vi "Test Host Image Acquisition Module Random Data.vi"(8 "error in":errorcluster, 11 "Operation":T3) -> (0 "error out":errorcluster, 1 "Image Acquired":bool, 2 "Acq In Progress":bool, 3 "Image":T2(plugin-control))   [LabVIEW 2013]
uses:
  Host/Image Acquisition/Host Image Acquisition Module Enum.ctl
  Host/Image Acquisition/Acquisition Settings Cluster.ctl
  <vilib>/vision/Image Controls.llb/IMAQ Image.ctl
  Host/Image Acquisition/Image Acquisition Settings FG Enum.ctl
  Host/System Status/Status FG Enum.ctl
  Host/Image Processing/Mask ROI FG Enum.ctl
  <vilib>/FPGAPlugInAG/PCIe-7842R/niLvFpga_Reset_PCIe-7842R.vi
  <vilib>/Utility/error.llb/Error Cluster From Error Code.vi
  <vilib>/rvi/errors/niLvFpgaAdjustHostInterfaceError.vi
  <vilib>/FPGAPlugInAG/PCIe-7842R/niLvFpga_Run_PCIe-7842R.vi
  <vilib>/FPGAPlugInAG/PCIe-7842R/niLvFpga_Close_PCIe-7842R.vi
  <vilib>/rvi/interface/nirviMethod/nirviMethod.xnode
  Host/FGs/FPGA_Reference.ctl
  FPGA Bitfiles/WingBeatAnalyzer_FPGATargetSim_10_2.lvbitx
  <vilib>/rvi/interface/nirviReadWriteControl/nirviReadWriteControl.xnode
  Common/CL Configuration.ctl
  Common/CL Signal Mapping.ctl
  FPGA/Sector/Accumulate/Sector Parameter Cluster.ctl
  <vilib>/rvi/interface/nirviCloseFPGA/nirviCloseFPGA.xnode
  Common/Timing/Timing Lib.lvlib
  Host/Globals/Average Sector Data.vi
  <vilib>/rvi/errors/niLvFpgaMergeErrorWithErrorCode.vi
  NiFpgaLv.dll
  <vilib>/FPGAPlugInAG/PCIe-7842R/niLvFpga_ReadFifo_PCIe-7842R.vi
  <vilib>/FPGAPlugInAG/PCIe-7842R/niLvFpga_ConfigureFifo_PCIe-7842R.vi
  <vilib>/FPGAPlugInAG/PCIe-7842R/niLvFpga_StartFifo_PCIe-7842R.vi
panel:
  out "Number of Elements to Write Sector Grouping FIFO":u32
  out "Actual Depth":u32
  out "Target Sim TO":bool
  out "Cam Data Timeout":bool
  out "Sector FIFO Timeout":bool
  out "Host DMA Timeout":bool
  out "Number of Elements to Write Host DMA":u32
  out "Number of Elements to Read Cam Data":u32
  out "Words per image":u32
  out "Num Frames read":u32
  out "DMA Words per Image":u32
  out "Acquire":bool
  in  "Acquisition Settings Cluster":T1={"Image Width"=2040, "Image Height"=1088, "Frames To Acquire"=0, "Signal Mapping"=enum."Basler 10-tap", "DMA Buffer Size\n(In Images)"=64} {"Image Height" max=65535; "Image Width" max=65535 step=40}
  out "Buffer Size":u32
  out "Acq'd Frame Width":u32=2040
  out "DMA Write Timeout":bool
  in  "Start Serial Server":bool
  out "Frames Acq'd":u32=1
  out "Acq'd Frame Height":u32=1088
  out "Initialized":bool
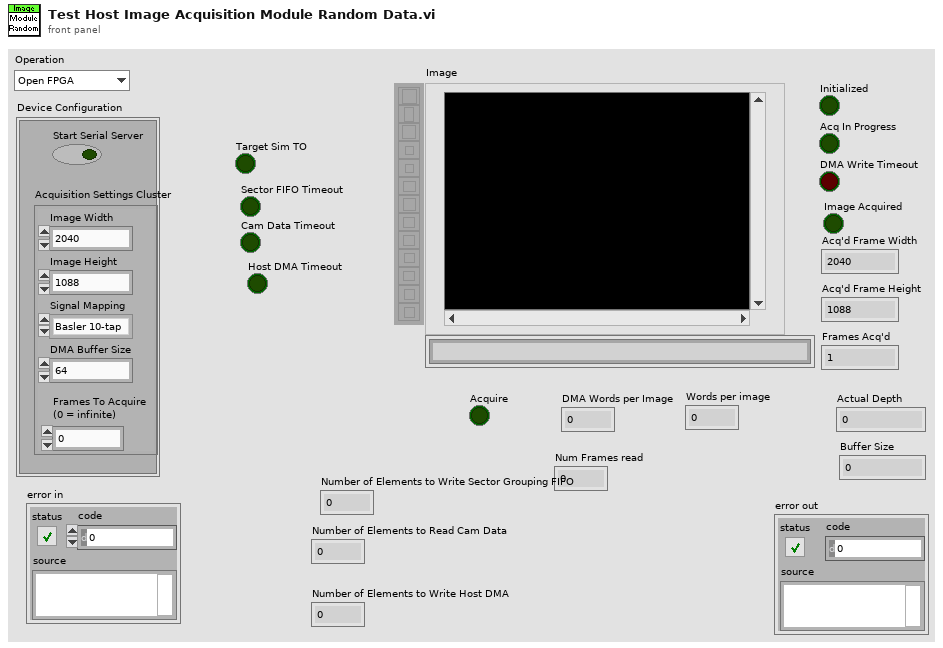
[diagram p1: front panel]
types:
  T1 = typedef "Acquisition Settings Cluster.ctl" = cluster{"Image Width":u32, "Image Height":u32, "Frames To Acquire":u32, "Signal Mapping":enum8{"Standard", "Basler 10-tap", "Vosskühler 10-tap"}, "DMA Buffer Size\n(In Images)":u32}
  T2 = typedef "IMAQ Image.ctl" = refnum<image>
  T3 = typedef "Host Image Acquisition Module Enum.ctl" = enum16{"Open FPGA", "Initialize DMA FIFO", "Load Sim Images", "Initialize Acquisition", "Update Sector Parameters", "Start Acquisition", "Aquire Image", "Read Averages", "Cancel Acquisition", "Close FPGA"}
  T4 = enum8{"Standard", "Basler 10-tap", "Vosskühler 10-tap"}
  T5 = typedef "Image Acquisition Settings FG Enum.ctl" = enum16{"Read", "Write"}
  T6 = typedef "Status FG Enum.ctl" = enum16{"Reset", "Read", "Write"}
  T7 = typedef "Mask ROI FG Enum.ctl" = enum16{"Read", "Write"}
  T8 = typedef "FPGA_Reference.ctl" = refnum<k20>
  T9 = typedef "Image Type" = u32
  T10 = typedef "Mask ROI Cluster.ctl" = cluster{"left annulus":T11, "right annulus":T11, "Threshold Range":cluster{"Lower value":dbl, "Upper value":dbl}, "[Avg BG]":u8[], "Number of Sectors":u8, "Left ROI":T12, "Right ROI":T12, "Left Start Angle Duty Cycle":fxp<+,8,0>, "Left End Angle Duty Cycle":fxp<+,8,0>, "Right End Angle Duty Cycle":fxp<+,8,0>, "Right Start Angle Duty Cycle":fxp<+,8,0>, "[Sector ROIs]":T12[]}
  T11 = typedef "IMAQ Circle" = cluster{"Center X":i32, "Center Y":i32, "Inner Radius":i32, "Outer Radius":i32, "Start Angle":dbl, "End Angle":dbl}
  T12 = typedef "ROI Descriptor" = cluster{"Global Rectangle":i32[], "Contours":cluster{"ID":enum32{"External", "Internal"}, "Type":u32, "Coordinates":i32[]}[]}
  T13 = typedef "Sector Parameter Cluster.ctl" = cluster{"Start Angle":fxp<+/-,17,2>, "End Angle":fxp<+,17,3>, "Inner Radius":u16, "Outter Radius":u16, "Hinge X":u16, "Hinge Y":u16, "NumWingSectors":u8}
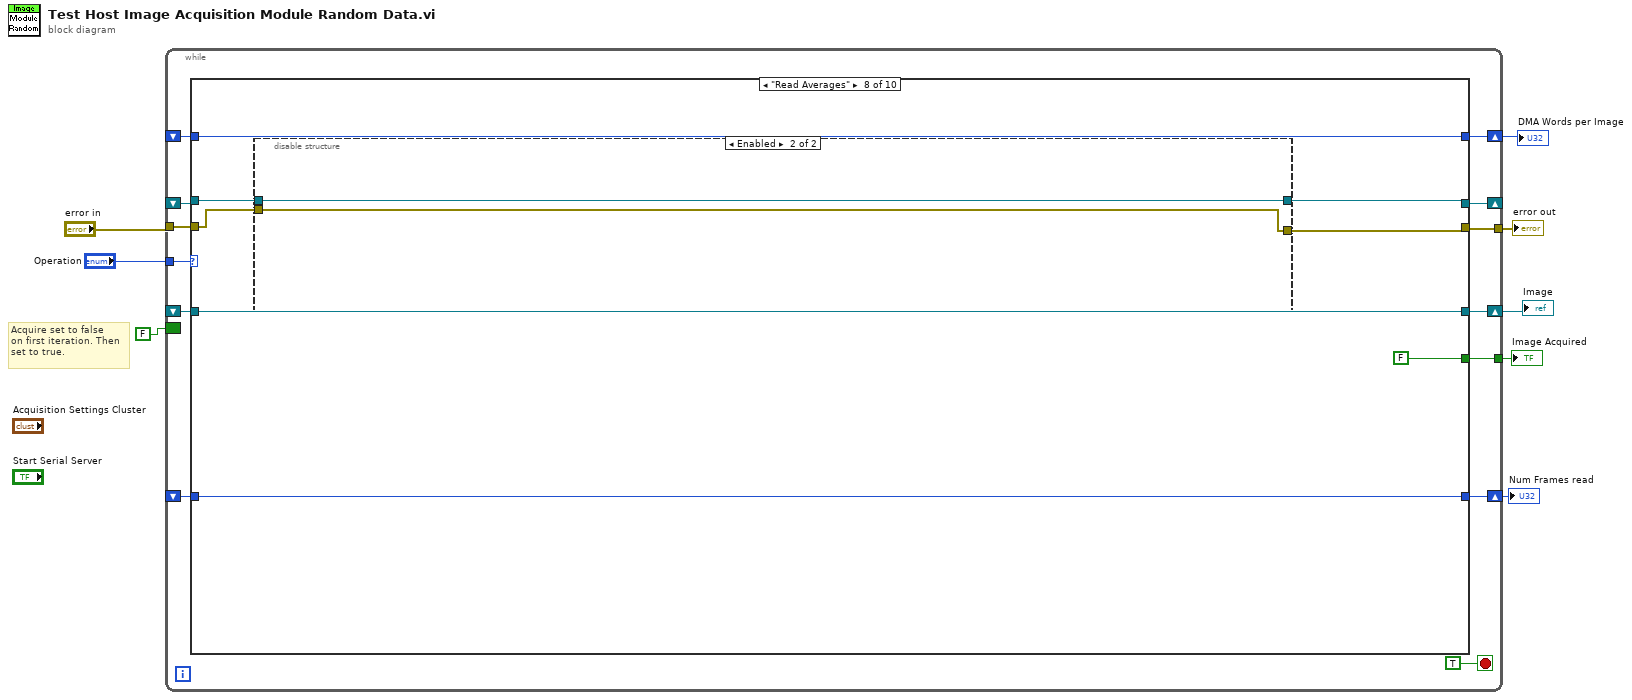
[diagram p0: block diagram]
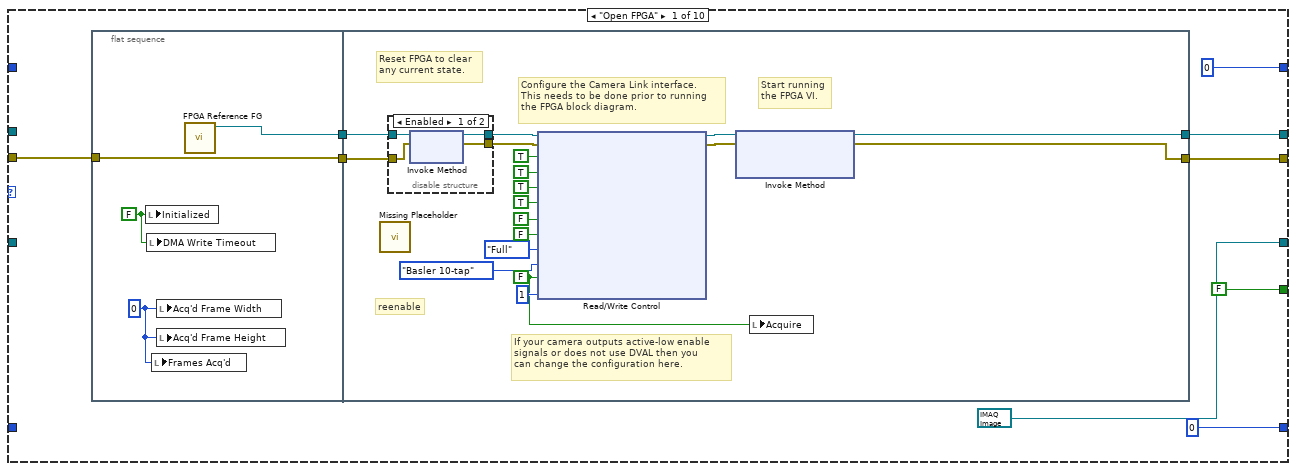
[diagram p2: hidden frame]
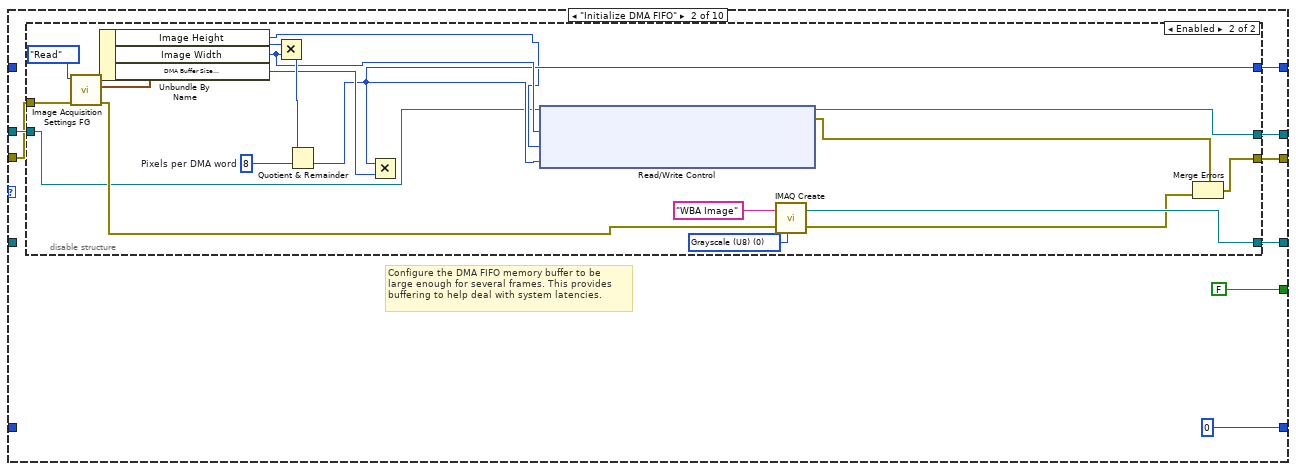
[diagram p4: hidden frame]
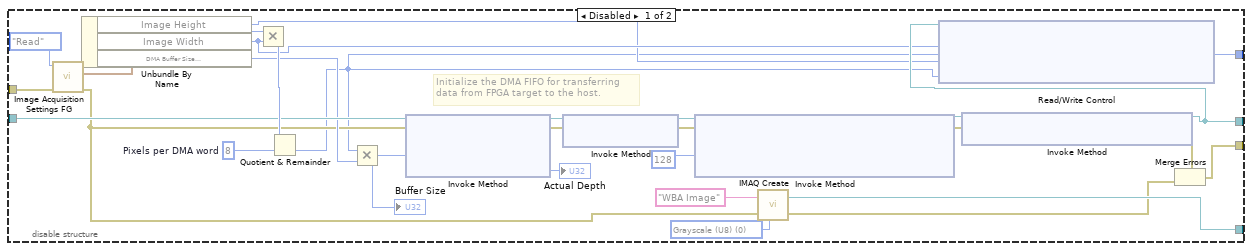
[diagram p5: hidden frame]
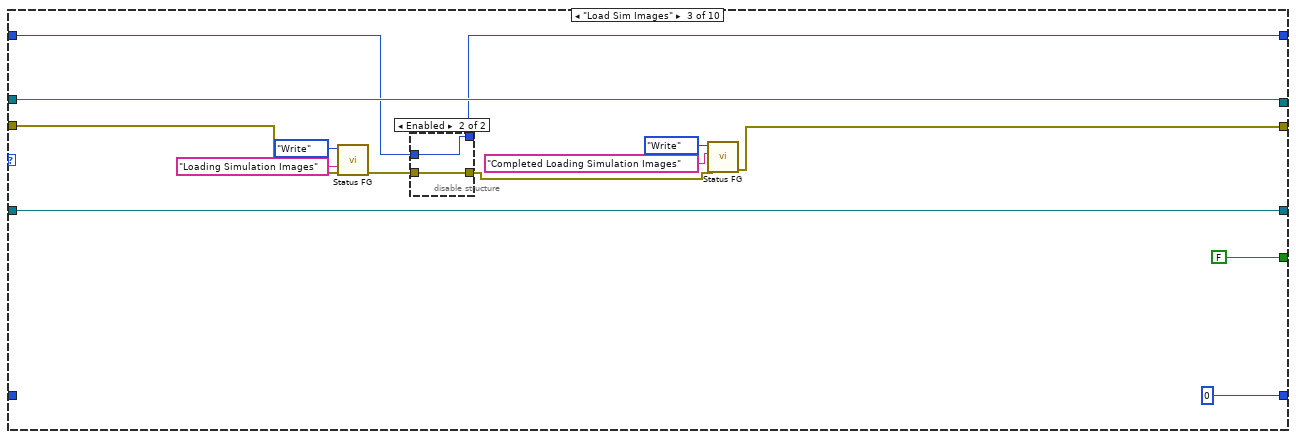
[diagram p6: hidden frame]
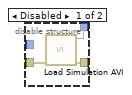
[diagram p7: hidden frame]
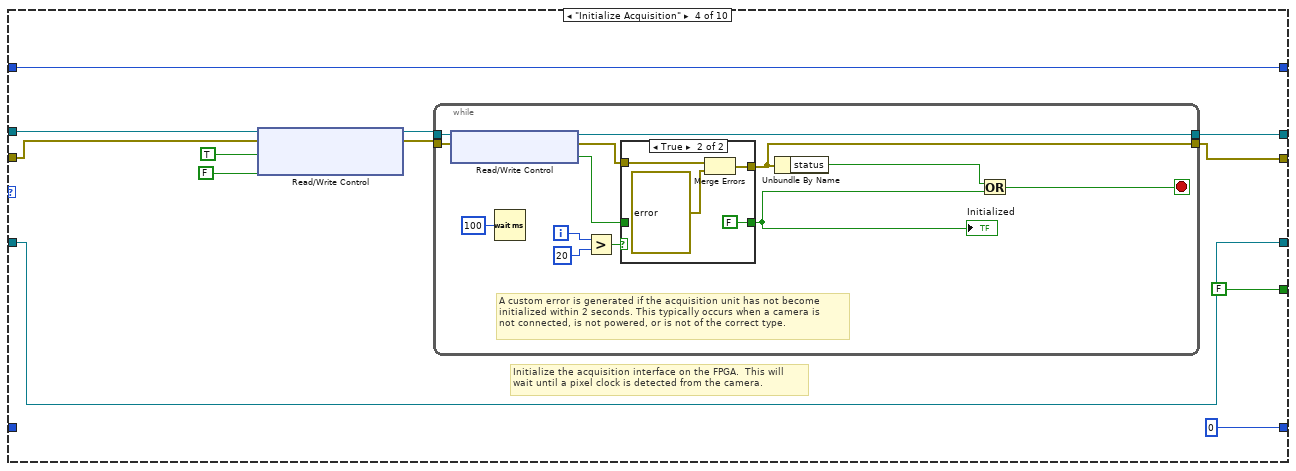
[diagram p8: hidden frame]
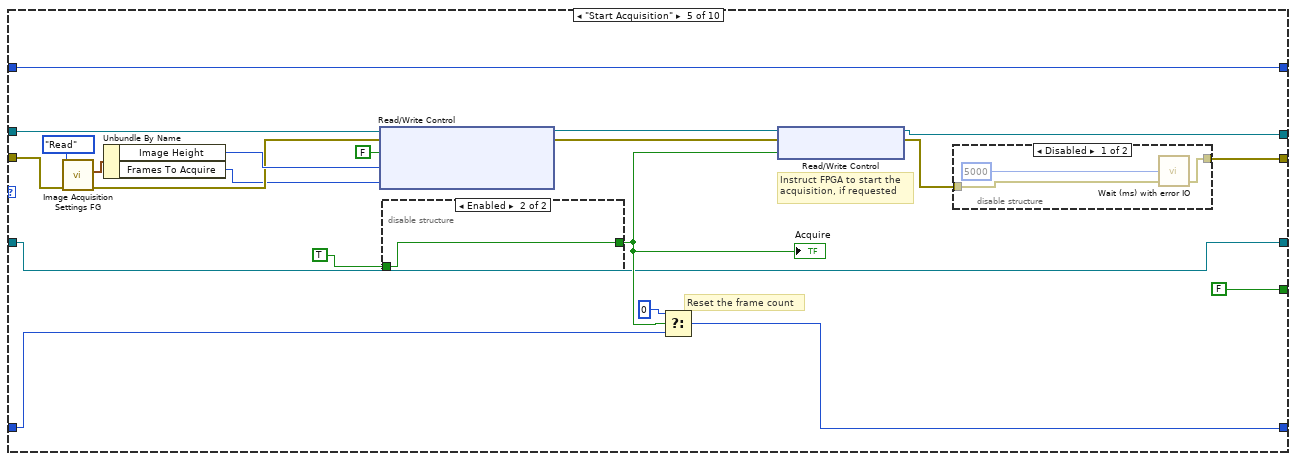
[diagram p10: hidden frame]
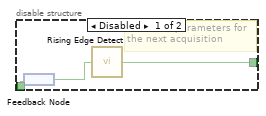
[diagram p12: hidden frame]
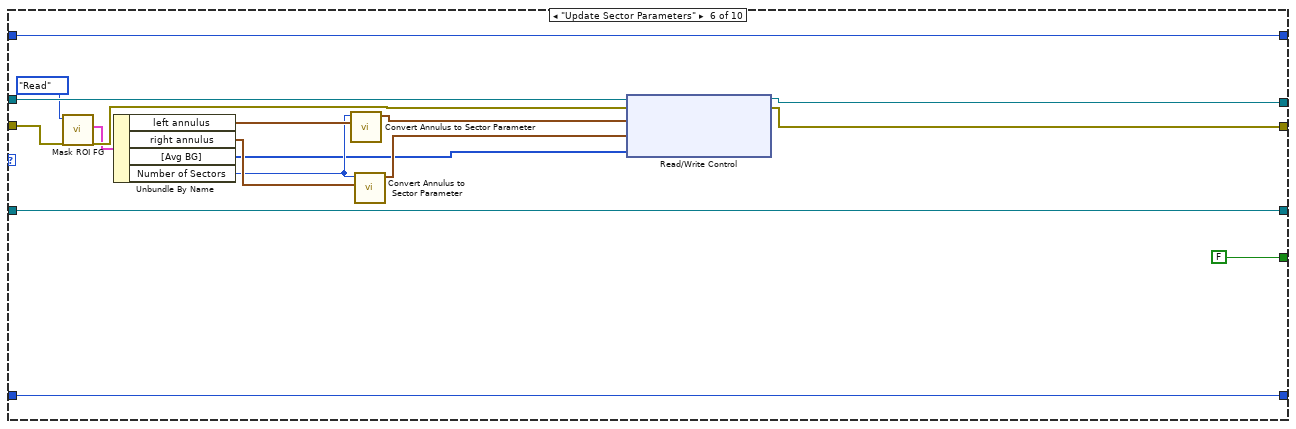
[diagram p13: hidden frame]
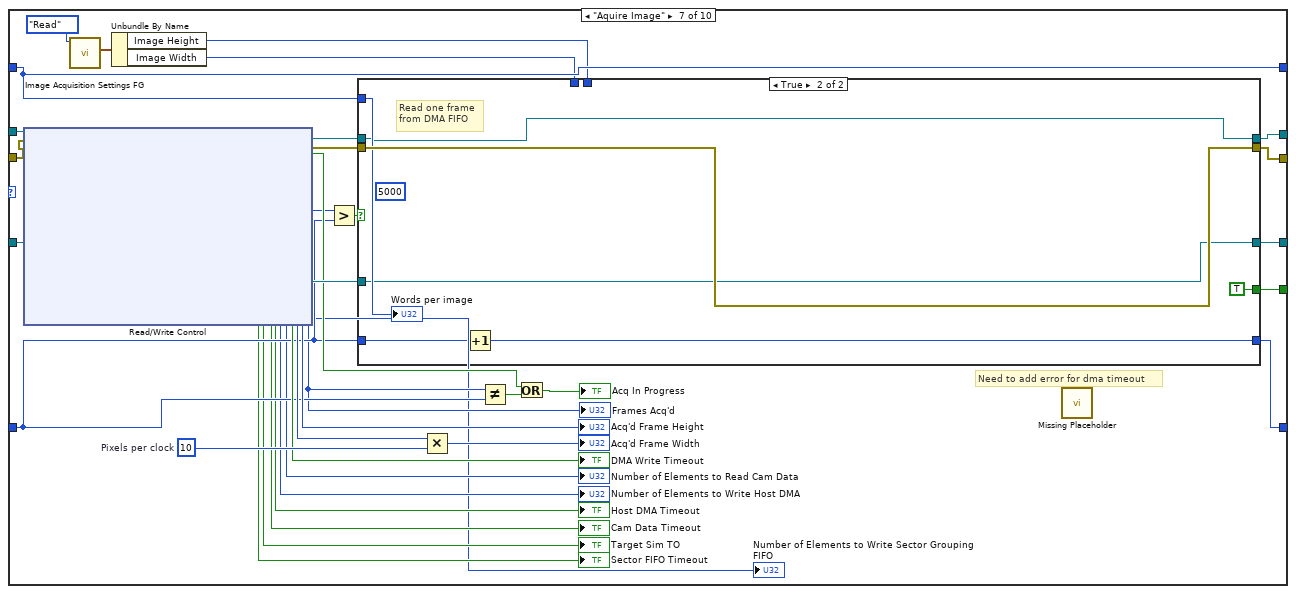
[diagram p14: hidden frame]
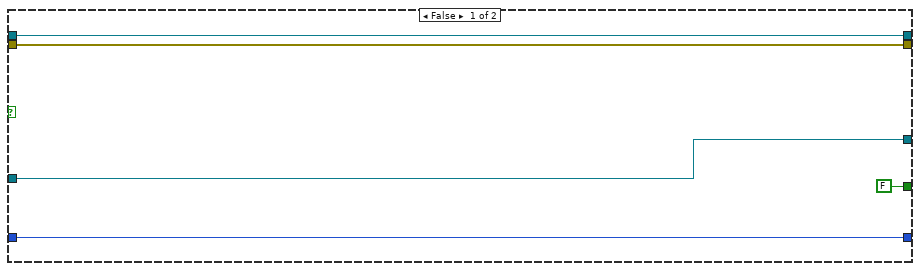
[diagram p15: hidden frame]
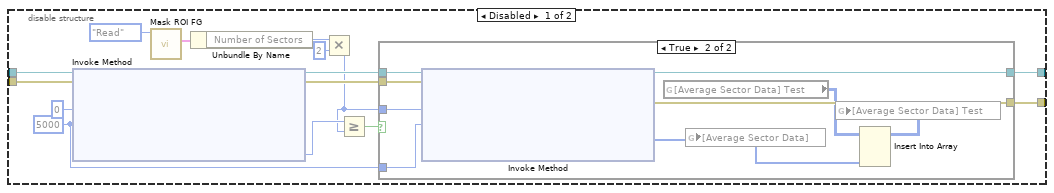
[diagram p16: hidden frame]
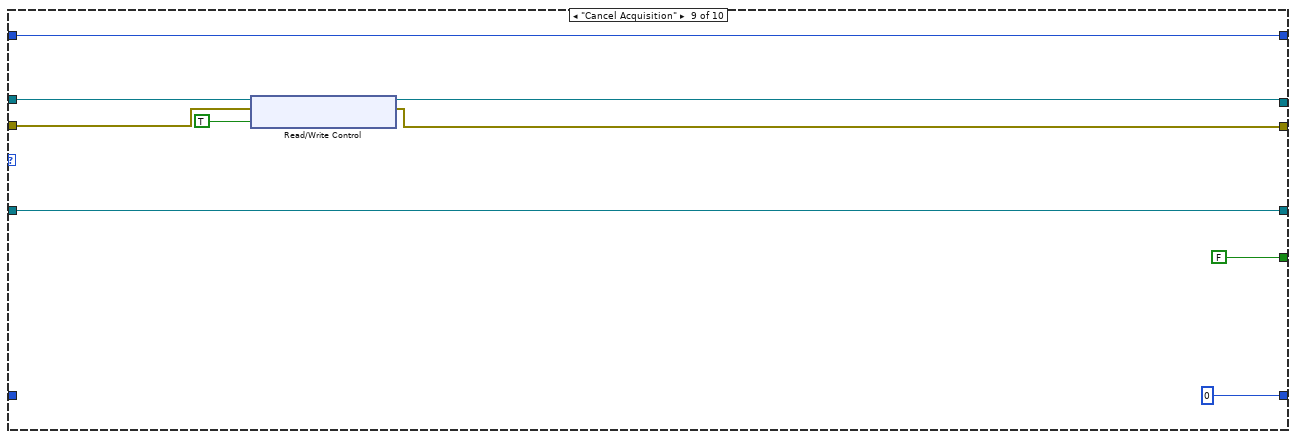
[diagram p18: hidden frame]
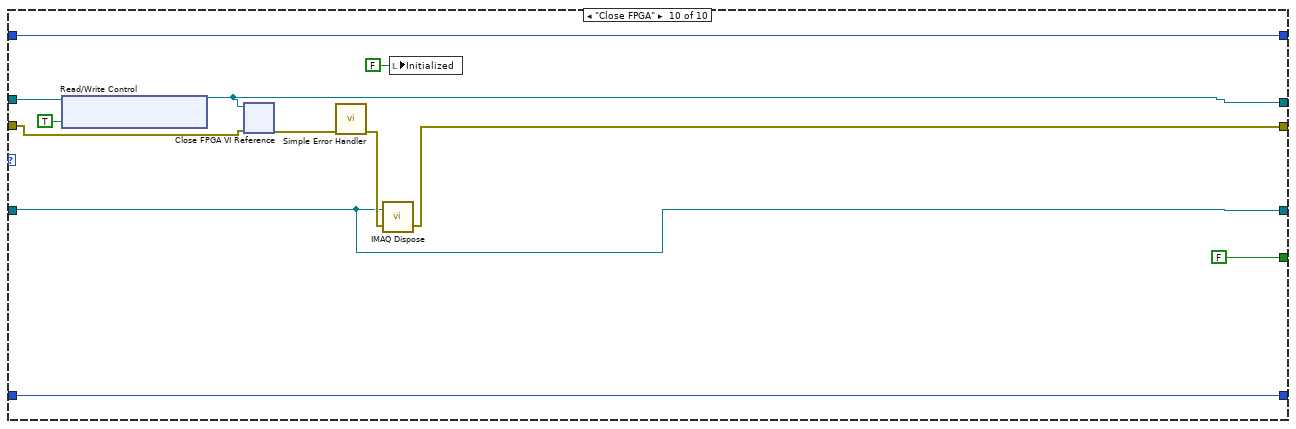
[diagram p19: hidden frame]
diagram:
  # "Acquire set to false\non first iteration. Then\nset to true."
  n1 = while {
    shift-right: [w20] -> _
    shift-left: _ -> [w16]
    tunnel: "error in" -> [w19]
    tunnel: "Operation" -> [w18]
    tunnel: [w17] -> w6
    shift-right: [w15] -> w3
    shift-left: _ -> [w14]
    shift-right: [w13] -> w4
    shift-left: _ -> [w10]
    shift-right: [w12] -> w2
    shift-left: _ -> [w11]
    border: FALSE ("Acquire") -> [_]
    tunnel: [w9] -> w1
    stop <- TRUE stop-if-true
    n2 = case shown="\"Read Averages\"" w18 {
      tunnel: w19 -> [w30 w63 w120 w132 w175 w205 w221 w253 w293 w299]
      tunnel: [w29 w60 w123 w138 w168 w201 w239 w259 w295 w300] -> w20
      tunnel: [w28 w62 w114 w134 w166 w202 w238 w254 w292 w306] -> w17
      tunnel: w16 -> [_ w66 w123 w139 w176 w207 w240 w260 w297 w302]
      tunnel: [u32 0 w59 w122 w137 w171 w206 w231 w258 w291 w303] -> w15
      tunnel: w14 -> [_ _ w112 w137 w171 w206 w231 w258 w291 w303]
      tunnel: [T2 refnum ("New Image") w64 w124 w133 w170 w192 w233 w257 w294 w304] -> w13
      tunnel: [u32 0 u32 0 u32 0 u32 0 w172 w200 w237 w256 u32 0 w305] -> w12
      tunnel: w11 -> [_ _ _ _ w173 w200 w219 w256 _ w305]
      tunnel: w10 -> [_ _ w124 w133 w170 w192 w232 w257 w294 w304]
      tunnel: [FALSE ("Image Acquired") FALSE ("Image Acquired") FALSE ("Image Acquired") FALSE ("Image Acquired") FALSE ("Image Acquired") FALSE ("Image Acquired") w213 FALSE ("Image Acquired") FALSE ("Image Acquired") FALSE ("Image Acquired")] -> w9
      frame "Open FPGA" {
        n3 = flat-sequence {
          tunnel: w30 -> [w31]
          tunnel: [w32] -> w27
          tunnel: [w31] -> w26
          tunnel: [w37] -> w28
          tunnel: [w38] -> w29
          tunnel: w27 -> [w42]
          tunnel: w26 -> [w39]
          frame #0 {
            w33 = u32 0 ("Acq'd Frame Width")
            w34 = FALSE ("Initialized")
            n4 = local write "Initialized"(w34) -> ()
            n5 = local write "DMA Write Timeout"(w34) -> ()
            n6 = local write "Frames Acq'd"(w33) -> ()
            n7 = local write "Acq'd Frame Width"(w33) -> ()
            n8 = local write "Acq'd Frame Height"(w33) -> ()
            n9 = call "FPGA Reference FG.vi"() -> ("FPGA VI Reference Out"=w32:T8)  [unwired: 11 in]
          }
          frame #1 {
            w35 = FALSE ("Acq Control.Acquire")
            # "reenable"
            # "If your camera outputs active-low enable\nsignals or does not use DVAL then you \ncan change the configuration here."
            # "Start running\nthe FPGA VI."
            # "Reset FPGA to clear\nany current state."
            # "Configure the Camera Link interface.\nThis needs to be done prior to running\nthe FPGA block diagram."
            n10 = call "Missing Placeholder.vi"() -> ()  [unwired: 12 in]
            n11 = disable-structure shown="Enabled" {
              disable-tunnel: [w56 w58] -> w46
              disable-tunnel: [w55 w57] -> w44
              disable-tunnel: w42 -> [w54 w58]
              disable-tunnel: w39 -> [w53 w57]
              frame Enabled {
                n12 = xnode "Invoke Method"("FPGA VI Reference In"=w54, "error in"=w53) -> ("FPGA VI Reference Out"=w56:T8, "error out"=w55:errorcluster)
              }
              frame Disabled {
              }
            }
            n13 = xnode "Read/Write Control"("FPGA VI Reference In"=w46, "error in"=w44, "CL Config.FVAL Active High"=TRUE ("IO Module Config.CL FVAL Active High"), "CL Config.LVAL Active High"=TRUE ("IO Module Config.CL LVAL Active High"), "CL Config.DVAL Active High"=TRUE ("IO Module Config.CL DVAL Active High"), "CL Config.Spare Active High"=TRUE ("IO Module Config.CL Spare Active High"), "CL Config.Line Scan"=FALSE, "Acq Control.Ignore DVAL"=FALSE ("CL Config.Line Scan"), "CL Config.Configuration"=enum8{"Base", "Medium", "Full"}."Full", "CL Config.Signal Mapping"=T4."Basler 10-tap", "Acq Control.Acquire"=w35, "# of Frames to Average"=u8 1) -> ("FPGA VI Reference Out"=w43:T8, "error out"=w45:errorcluster)
            n14 = xnode "Invoke Method"("FPGA VI Reference In"=w43, "error in"=w45) -> ("FPGA VI Reference Out"=w38:T8, "error out"=w37:errorcluster)  [unwired: 1 in]
            n15 = local write "Acquire"(w35) -> ()
          }
        }
      }
      frame "Initialize DMA FIFO" {
        # "Configure the DMA FIFO memory buffer to be\nlarge enough for several frames. This provides\nbuffering to help deal with system latencies."
        n16 = disable-structure shown="Enabled" {
          disable-tunnel: w66 -> [w88 w94]
          disable-tunnel: [w85 w107] -> w64
          disable-tunnel: w63 -> [w82 w104]
          disable-tunnel: [w74 w100] -> w62
          disable-tunnel: [w70 w98] -> w60
          disable-tunnel: [w67 w96] -> w59
          frame Disabled {
            w86 = T9 0 items=["Grayscale (U8)", "Grayscale (I16)", "Grayscale (SGL)", "Complex (CSG)", "RGB (U32)", "HSL (U32)", "RGB (U64)", "Grayscale (U16)"] ("Image Type")
            w90 = u32 8  # Pixels per DMA word
            # "Initialize the DMA FIFO for transferring\ndata from FPGA target to the host."
            n17 = call "Image Acquisition Settings FG.vi"("error in (no error)"=w82, "Operation"=Image_Acquisition_Settings_FG_Enum."Read") -> ("error out"=w77:errorcluster, "Acquisition Settings Out"=w83:T1)  [unwired: 8 in]
            n18 = Unbundle By Name(w83) -> ("Image Height"=w68:u32, "Image Width"=w69:u32, "DMA Buffer Size\n(In Images)"=w81:u32)
            n19 = Multiply(x=w68, y=w69) -> (x*y=w89:u32)
            n20 = Quotient & Remainder(x=w89, y=w90) -> (floor(x/y)=w67:u32)  [unwired: 1 out]
            n21 = Multiply(x=w67, y=w81) -> (x*y=w91:u32)
            "Buffer Size" <- w91
            n22 = xnode "Invoke Method"("FPGA VI Reference In"=w88, "error in"=w77, "Requested Depth"=w91) -> ("FPGA VI Reference Out"=w93:T8, "error out"=w92:errorcluster, "Actual Depth"=→"Actual Depth":u32)
            n23 = xnode "Invoke Method"("FPGA VI Reference In"=w93, "error in"=w92) -> ("FPGA VI Reference Out"=w73:T8, "error out"=w71:errorcluster)
            n24 = xnode "Invoke Method"("FPGA VI Reference In"=w73, "error in"=w71, "Requested Depth"=u32 128) -> ("FPGA VI Reference Out"=w79:T8, "error out"=w78:errorcluster)  [unwired: 1 out]
            n25 = call "IMAQ Create"("Image Name"="WBA Image", "Image Type"=w86, "error in (no error)"=w77) -> ("New Image"=w85:T2, "error out"=w76:errorcluster)  [unwired: 2 in]
            n26 = xnode "Invoke Method"("FPGA VI Reference In"=w79, "error in"=w78) -> ("FPGA VI Reference Out"=w70:T8, "error out"=w75:errorcluster)
            n27 = xnode "Read/Write Control"("FPGA VI Reference In"=w70, "X Resolution"=w69, "Y Resolution"=w68, "Words per image"=w67) -> ()  [unwired: 1 in, 2 out]
            n28 = Merge Errors(w75, w76) -> (w74:errorcluster)
          }
          frame Enabled {
            w108 = T9 0 items=["Grayscale (U8)", "Grayscale (I16)", "Grayscale (SGL)", "Complex (CSG)", "RGB (U32)", "HSL (U32)", "RGB (U64)", "Grayscale (U16)"] ("Image Type")
            w111 = u32 8  # Pixels per DMA word
            n29 = call "Image Acquisition Settings FG.vi"("error in (no error)"=w104, "Operation"=Image_Acquisition_Settings_FG_Enum."Read") -> ("error out"=w102:errorcluster, "Acquisition Settings Out"=w105:T1)  [unwired: 8 in]
            n30 = Unbundle By Name(w105) -> ("Image Height"=w95:u32, "Image Width"=w99:u32, "DMA Buffer Size\n(In Images)"=w103:u32)
            n31 = Multiply(x=w95, y=w99) -> (x*y=w110:u32)
            n32 = Quotient & Remainder(x=w110, y=w111) -> (floor(x/y)=w96:u32)  [unwired: 1 out]
            n33 = Multiply(x=w96, y=w103) -> ()  [unwired: 1 out]
            n34 = xnode "Read/Write Control"("FPGA VI Reference In"=w94, "X Resolution"=w99, "Y Resolution"=w95, "Words per image"=w96) -> ("FPGA VI Reference Out"=w98:T8, "error out"=w97:errorcluster)  [unwired: 1 in]
            n35 = call "IMAQ Create"("Image Name"="WBA Image", "Image Type"=w108, "error in (no error)"=w102) -> ("New Image"=w107:T2, "error out"=w101:errorcluster)  [unwired: 2 in]
            n36 = Merge Errors(w97, w101) -> (w100:errorcluster)
          }
        }
      }
      frame "Load Sim Images" {
        n37 = call "Status FG.vi"("error in (no error)"=w120, "Status In"="Loading Simulation Images", "Operation"=Status_FG_Enum."Write") -> ("error out"=w119:errorcluster)  [unwired: 7 in, 1 out]
        n38 = disable-structure shown="Enabled" {
          disable-tunnel: [w128 w129] -> w122
          disable-tunnel: w119 -> [w127 w130]
          disable-tunnel: [w126 w130] -> w115
          disable-tunnel: w112 -> [_ w129]
          frame Disabled {
            n39 = call "Load Simulation AVI.vi"("error in (no error)"=w127) -> ("error out"=w126:errorcluster, "Words per image"=w128:u32)  [unwired: 9 in]
          }
          frame Enabled {
          }
        }
        n40 = call "Status FG.vi"("error in (no error)"=w115, "Status In"="Completed Loading Simulation Images", "Operation"=Status_FG_Enum."Write") -> ("error out"=w114:errorcluster)  [unwired: 7 in, 1 out]
      }
      frame "Initialize Acquisition" {
        # "Initialize the acquisition interface on the FPGA.  This will\nwait until a pixel clock is detected from the camera."
        n41 = xnode "Read/Write Control"("FPGA VI Reference In"=w139, "error in"=w132, "Acq Control.Initialize"=TRUE ("Arm Acquisition"), "Acq Control.Cancel Acq"=FALSE) -> ("FPGA VI Reference Out"=w142:T8, "error out"=w141:errorcluster)
        n42 = while {
          tunnel: w142 -> [w151]
          tunnel: w141 -> [w150]
          tunnel: [w149] -> w138
          tunnel: [w152] -> w134
          i -> [w145]
          stop <- w155 stop-if-true
          # "A custom error is generated if the acquisition unit has not become\ninitialized within 2 seconds. This typically occurs when a camera is\nnot connected, is not powered, or is not of the correct type."
          n43 = xnode "Read/Write Control"("FPGA VI Reference In"=w151, "error in"=w150) -> ("FPGA VI Reference Out"=w149:T8, "error out"=w148:errorcluster, "Acq Status.Initialized"=w147:bool)
          n44 = Wait (ms)(milliseconds to wait=u32 100) -> ()  [unwired: 1 out]
          n45 = Greater?(x=w145, y=20) -> (0:w146:bool)
          n46 = case shown="True" w146 {
            tunnel: [w157 FALSE] -> w143
            tunnel: w147 -> [w157 _]
            tunnel: w148 -> [w156 w159]
            tunnel: [w156 w161] -> w152
            frame False {
            }
            frame True {
              n47 = Merge Errors(w159, errorcluster {"status"=TRUE, "code"=-8999, "source"="Acquisition Initialization: This error typically occurs when a camera is not properly connected, is not powered, or is not of the correct type."} ("error in")) -> (w161:errorcluster)
            }
          }
          "Initialized" <- w143
          n48 = Unbundle By Name(w152) -> ("status"=w154:bool)
          n49 = Or(x=w154, y=w143) -> (x .or. y?=w155:bool)
        }
      }
      frame "Start Acquisition" {
        # "Reset the frame count"
        # "Instruct FPGA to start the\nacquisition, if requested"
        n50 = call "Image Acquisition Settings FG.vi"("error in (no error)"=w175, "Operation"=Image_Acquisition_Settings_FG_Enum."Read") -> ("error out"=w174:errorcluster, "Acquisition Settings Out"=w182:T1)  [unwired: 8 in]
        n51 = Unbundle By Name(w182) -> ("Image Height"=w177:u32, "Frames To Acquire"=w164:u32)
        n52 = xnode "Read/Write Control"("FPGA VI Reference In"=w176, "error in"=w174, "Acq Control.Cancel Acq"=FALSE, "Acq Control.Line Scan Height"=w177, "Acq Control.Frames To Acq"=w164) -> ("FPGA VI Reference Out"=w162:T8, "error out"=w163:errorcluster)
        n53 = disable-structure shown="Enabled" {
          disable-tunnel: [w189 w190] -> w179
          disable-tunnel: TRUE ("Acquire") -> [w187 w190]
          frame Disabled {
            # "Write the parameters for\nthe next acquisition"
            n54 = feedback #1() -> (w188:bool)
            n55 = feedback-in #1(w187) -> ()
            n56 = call "Rising Edge Detect.vi"("Input"=w188) -> ("Pulse"=w189:bool)  [unwired: 4 in]
          }
          frame Enabled {
          }
        }
        "Acquire" <- w179
        n57 = Select(t=u32 0, s=w179, f=w173) -> (s? t:f=w172:u32)
        n58 = xnode "Read/Write Control"("FPGA VI Reference In"=w162, "error in"=w163, "Acq Control.Acquire"=w179) -> ("FPGA VI Reference Out"=w168:T8, "error out"=w167:errorcluster)
        n59 = disable-structure shown="Disabled" {
          disable-tunnel: w167 -> [w184 w186]
          disable-tunnel: [w183 w186] -> w166
          frame Disabled {
            n60 = call "Wait (ms) with error IO.vi"("error in (no error)"=w184, "milliseconds to wait"=u32 5000) -> ("error out"=w183:errorcluster)  [unwired: 3 in]
          }
          frame Enabled {
          }
        }
      }
      frame "Update Sector Parameters" {
        n61 = call "Mask ROI FG.vi"("error in (no error)"=w205, "Operation"=Mask_ROI_FG_Enum."Read") -> ("error out"=w204:errorcluster, "Mask ROI Out"=w199:T10)  [unwired: 8 in]
        n62 = Unbundle By Name(w199) -> ("left annulus"=w198:T11, "right annulus"=w196:T11, "[Avg BG]"=w193:u8[], "Number of Sectors"=w195:u8)
        n63 = call "Convert Annulus to Sector Parameter.vi"("Annulus"=w198, "NumWingSectors"=w195) -> ("Sector Parameter"=w197:T13)  [unwired: 9 in]
        n64 = call "Convert Annulus to Sector Parameter.vi"("Annulus"=w196, "NumWingSectors"=w195) -> ("Sector Parameter"=w194:T13)  [unwired: 9 in]
        n65 = xnode "Read/Write Control"("FPGA VI Reference In"=w207, "error in"=w204, "Sector Parameters Left"=w197, "Sector Parameters Right"=w194, "[Average BG Intensity]"=w193) -> ("FPGA VI Reference Out"=w201:T8, "error out"=w202:errorcluster)
      }
      frame "Aquire Image" {
        w229 = u32 10  # Pixels per clock
        # "Need to add error for dma timeout"
        n66 = xnode "Read/Write Control"("FPGA VI Reference In"=w240, "error in"=w221) -> ("FPGA VI Reference Out"=w236:T8, "error out"=w235:errorcluster, "Acq Status.Acq In Progress"=w220:bool, "Acq Status.Frames Acq'd"=w218:u32, "Acq Status.Lines Per Frame"=→"Acq'd Frame Height":u32, "Acq Status.Clocks Per Line"=w228:u32, "Acq Status.DMA Write Timeout"=→"DMA Write Timeout":bool, "Number of Elements to Read Cam Data"=→"Number of Elements to Read Cam Data":u32, "Number of Elements to Write Host DMA"=→"Number of Elements to Write Host DMA":u32, "Host DMA Timeout"=→"Host DMA Timeout":bool, "Cam Data Timeout"=→"Cam Data Timeout":bool, "Target Sim TO"=→"Target Sim TO":bool, "Sector FIFO Timeout"=→"Sector FIFO Timeout":bool, "Number of Elements to Write Sector Grouping FIFO"=→"Number of Elements to Write Sector Grouping FIFO":u32)
        "Frames Acq'd" <- w218
        n67 = call "Image Acquisition Settings FG.vi"("Operation"=Image_Acquisition_Settings_FG_Enum."Read") -> ("Acquisition Settings Out"=w224:T1)  [unwired: 9 in, 1 out]
        n68 = Unbundle By Name(w224) -> ("Image Height"=w223:u32, "Image Width"=w222:u32)
        n69 = Greater?(x=w218, y=w219) -> (0:w234:bool)
        n70 = case shown="True" w234 {
          tunnel: w236 -> [w244 w246]
          tunnel: w235 -> [w243 w252]
          tunnel: w223 -> [_ _]
          tunnel: w222 -> [_ _]
          tunnel: w232 -> [w245 w248]
          tunnel: [w243 w252] -> w238
          tunnel: [w244 w246] -> w239
          tunnel: w219 -> [w242 w251]
          tunnel: [w242 w250] -> w237
          tunnel: w231 -> [_ w249]
          tunnel: [w245 w248] -> w233
          tunnel: [FALSE ("Image Acquired") TRUE ("Image Acquired")] -> w213
          frame False {
          }
          frame True {
            (unwired) 5000 ("Timeout (ms)")
            # "Read one frame\nfrom DMA FIFO"
            n71 = Increment(x=w251) -> (x+1=w250:u32)
            "Words per image" <- w249
          }
        }
        n72 = Multiply(x=w228, y=w229) -> (x*y=→"Acq'd Frame Width":u32)
        n73 = Not Equal?(x=w218, y=w219) -> (x != y?=w217:bool)
        n74 = Or(x=w220, y=w217) -> (x .or. y?=→"Acq In Progress":bool)
        n75 = call "Missing Placeholder.vi"() -> ()  [unwired: 12 in]
      }
      frame "Read Averages" {
        n76 = disable-structure shown="Enabled" {
          disable-tunnel: w260 -> [w275 w288]
          disable-tunnel: [w270 w288] -> w259
          disable-tunnel: [w269 w287] -> w254
          disable-tunnel: w253 -> [w267 w287]
          frame Disabled {
            w271 = 5000 ("Timeout (ms)")
            n77 = xnode "Invoke Method"("FPGA VI Reference In"=w275, "error in"=w267, "Number of Elements"=u32 0, "Timeout (ms)"=w271) -> ("FPGA VI Reference Out"=w273:T8, "error out"=w272:errorcluster, "Elements Remaining"=w263:u32)  [unwired: 1 out]
            n78 = call "Mask ROI FG.vi"("Operation"=Mask_ROI_FG_Enum."Read") -> ("Mask ROI Out"=w266:T10)  [unwired: 9 in, 1 out]
            n79 = Unbundle By Name(w266) -> ("Number of Sectors"=w264:u8)
            n80 = Multiply(x=w264, y=u8 2) -> (x*y=w262:u8)
            n81 = Greater Or Equal?(x=w263, y=w262) -> (x >= y?=w265:bool)
            n82 = case shown="True" w265 {
              tunnel: w273 -> [w277 w286]
              tunnel: w272 -> [w276 w285]
              tunnel: w271 -> [_ w284]
              tunnel: [w277 w283] -> w270
              tunnel: [w276 w282] -> w269
              tunnel: w262 -> [_ w281]
              frame False {
              }
              frame True {
                n83 = xnode "Invoke Method"("FPGA VI Reference In"=w286, "error in"=w285, "Number of Elements"=w281, "Timeout (ms)"=w284) -> ("FPGA VI Reference Out"=w283:T8, "error out"=w282:errorcluster, "Data"=w279:u8[])  [unwired: 1 out]
                n84 = global read "Average Sector Data.vi" "[Average Sector Data] Test"() -> (w280:u8[][])
                n85 = global write "Average Sector Data.vi" "[Average Sector Data]"(w279) -> ()
                n86 = Insert Into Array(array=w280, new element=w279) -> (w278:u8[][])  [unwired: 2 in]
                n87 = global write "Average Sector Data.vi" "[Average Sector Data] Test"(w278) -> ()
              }
            }
          }
          frame Enabled {
          }
        }
      }
      frame "Cancel Acquisition" {
        n88 = xnode "Read/Write Control"("FPGA VI Reference In"=w297, "error in"=w293, "Acq Control.Cancel Acq"=TRUE) -> ("FPGA VI Reference Out"=w295:T8, "error out"=w292:errorcluster)
      }
      frame "Close FPGA" {
        n89 = xnode "Read/Write Control"("FPGA VI Reference In"=w302, "Acq Control.Cancel Acq"=TRUE) -> ("FPGA VI Reference Out"=w300:T8)  [unwired: 1 in, 1 out]
        n90 = xnode "Close FPGA VI Reference"("FPGA VI Reference In"=w300, "error in"=w299) -> ("error out"=w309:errorcluster)
        n91 = call <vilib>:"Simple Error Handler.vi"("error in (no error)"=w309) -> ("error out"=w307:errorcluster)  [unwired: 4 in, 4 out]
        n92 = call "IMAQ Dispose"("Image"=w304, "error in (no error)"=w307) -> ("error out"=w306:errorcluster)  [unwired: 4 in]
        n93 = local write "Initialized"(FALSE ("Initialized")) -> ()
      }
    }
  }
  "error out" <- w6
  "Image" <- w4
  "DMA Words per Image" <- w3
  "Num Frames read" <- w2
  "Image Acquired" <- w1
